vi "ForceCurveSettings.vi"(0 "FPGA ref in":T2, 5 "Parameters":T1={"Start"=-1e-06, "Distance"=2e-07, "Points"=256.0, "Fwd"=0.0, "Bwd"=0.0, "Pause"=0.0} {"Pause" format="%#_3p"; "Bwd" format="%.0pm/s"; "Distance" format="%#.3pm"; "Start" format="%#.3pm"; "Fwd" format="%.0pm/s"}, 7 "Range Z":dbl, 9 "Bwd sweep":bool, 11 "error in":errorcluster, 12 "Points":dbl) -> (3 "BwdSweep(T=2, F=1)":dbl, 4 "FPGA ref out":T2, 6 "Zheight":dbl, 8 "PointsArray":dbl[](array[numeric]), 10 "RampDistancePoints":dbl[][](array[numeric]), 14 "Voltage Range":dbl, 15 "error out":errorcluster)   [LabVIEW 2016]
uses:
  controls/FPGAVIreferenceTypeDef.ctl
  controls/Enum.ctl
  <vilib>/Utility/error.llb/Error Cluster From Error Code.vi
  <vilib>/rvi/errors/niLvFpgaAdjustHostInterfaceError.vi
  <vilib>/rvi/interface/nirviReadWriteControl/nirviReadWriteControl.xnode
  FPGA Bitfiles/qnmController797_usbRIO_controllerFPGAmu.lvbitx
  NiFpgaLv.dll
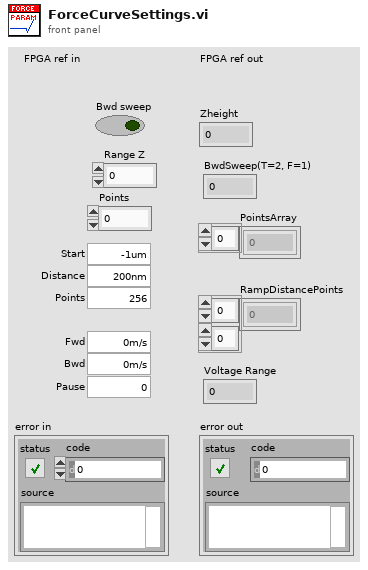
[diagram p1: front panel]
types:
  T1 = cluster{"Start":dbl, "Distance":dbl, "Points":dbl, "Fwd":dbl, "Bwd":dbl, "Pause":dbl}
  T2 = typedef "FPGAVIreferenceTypeDef.ctl" = refnum<k20>
  T3 = typedef "Enum.ctl" = enum16{"Init", "Read", "Write"}
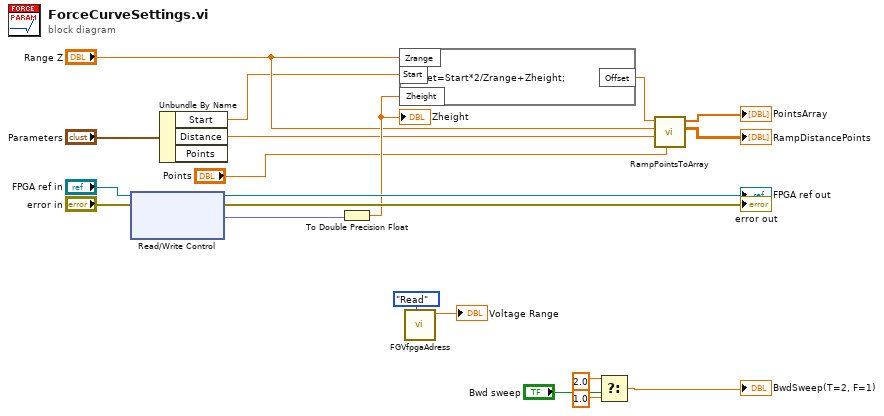
[diagram p0: block diagram]
diagram:
  n1 = xnode "Read/Write Control"("FPGA VI Reference In"="FPGA ref in", "error in"="error in") -> ("FPGA VI Reference Out"=→"FPGA ref out":T2, "error out"=→"error out":errorcluster, "fb.o.height"=w9:fxp<+/-,31,4>)  [unwired: 1 out]
  n2 = Unbundle By Name("Parameters") -> ("Start"=w8:dbl, "Distance"=w11:dbl)  [unwired: 1 out]
  n3 = To Double Precision Float(number=w9) -> (double precision float=w15:dbl)
  "Zheight" <- w15
  n4 = formula code="Offset=Start*2/Zrange+Zheight;"("Start"=w8, "Zheight"=w15, "Zrange"="Range Z") -> ("Offset"=w10:dbl)
  n5 = call "FGVfpgaAdress.vi"("Enum"=Enum."Read") -> ("voltageRange(+/-)Out"=→"Voltage Range":dbl)  [unwired: 5 in, 5 out]
  n6 = Select(t=2.0 ("y"), s="Bwd sweep", f=1.0 ("y")) -> (s? t:f=→"BwdSweep(T=2, F=1)":dbl)
  n7 = call "RampPointsToArray.vi"("Points"="Points", "Distance"=w11, "Range Z"="Range Z", "Offset"=w10) -> ("RampDistancePoints"=→"RampDistancePoints":dbl[][], "PointsArray"=→"PointsArray":dbl[])  [unwired: 6 in]
